vi "João aula 5.vi"() -> ()   [LabVIEW 2024]
uses:
  <vilib>/LabVIEW Open Source Project/Epoch Date & Time/epoch.UNIX/Epoch.UNIX.lvclass
panel:
  out "Potencia ativa C":waveform(dbl)(graph)
  out "Potencia ativa C":waveform(dbl)(graph)
  out "Potencia ativa C":waveform(dbl)
  out "Potencia ativa B":waveform(dbl)(graph)
  out "Potencia ativa B":waveform(dbl)(graph)
  out "Potencia ativa B":waveform(dbl)
  out "Potencia ativa A":waveform(dbl)(graph)
  out "Potencia ativa A":waveform(dbl)(graph)
  in  "stop":bool
  out "Potencia ativa A":waveform(dbl)
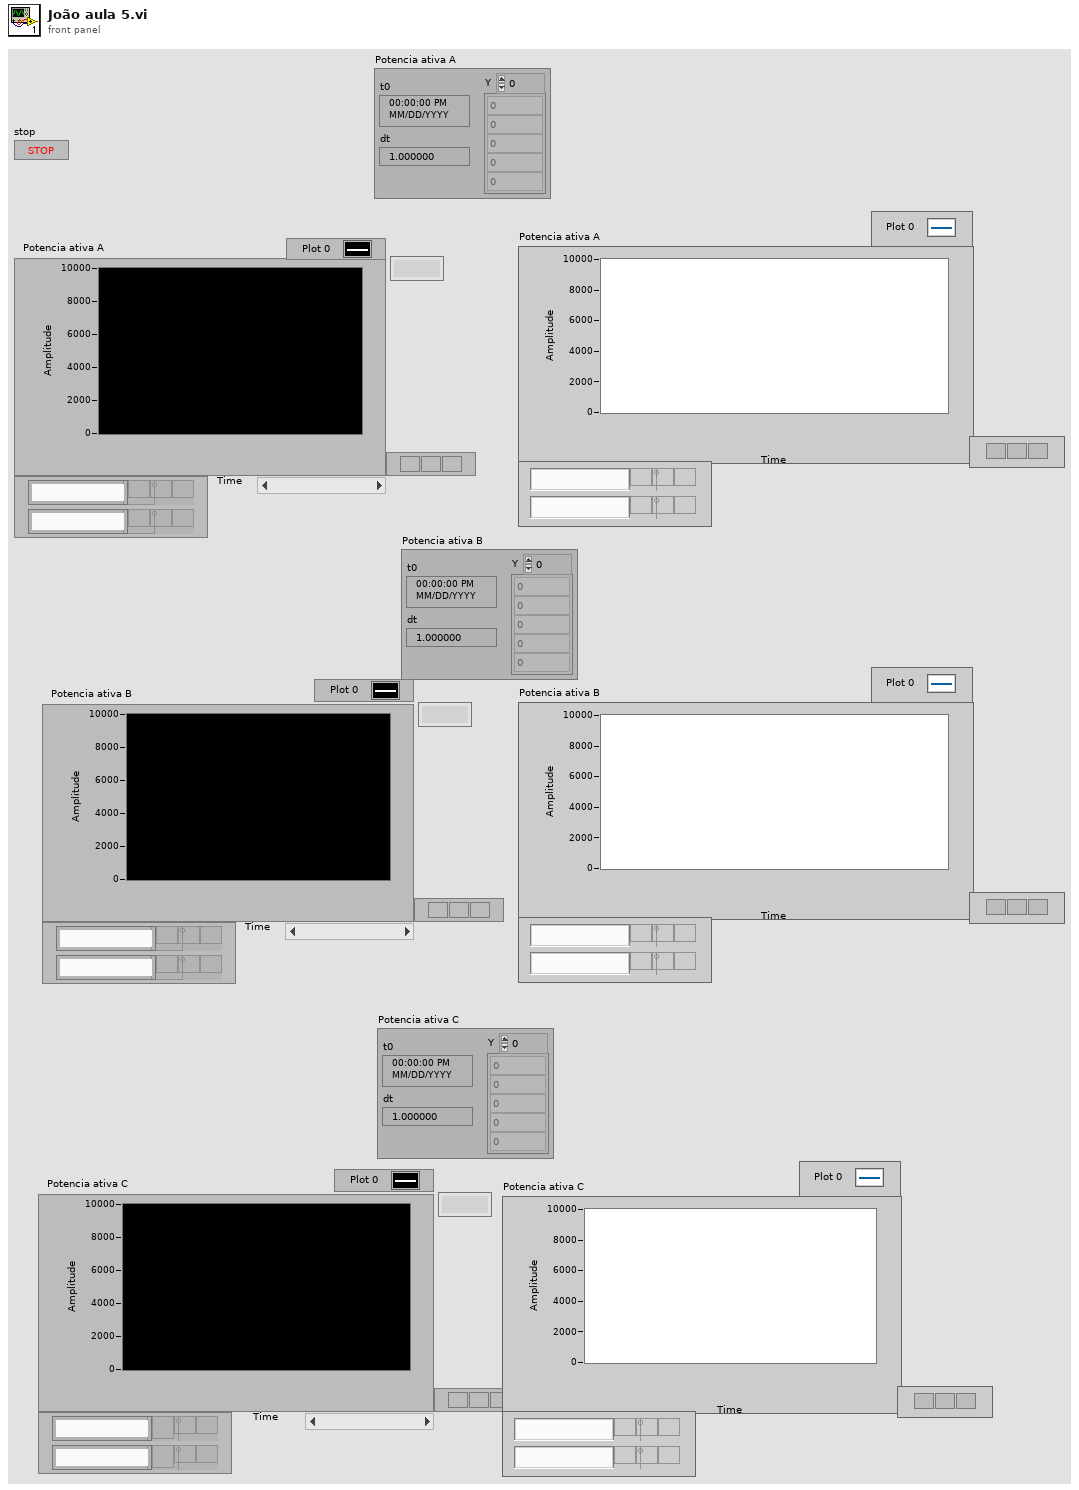
[diagram p1: front panel]
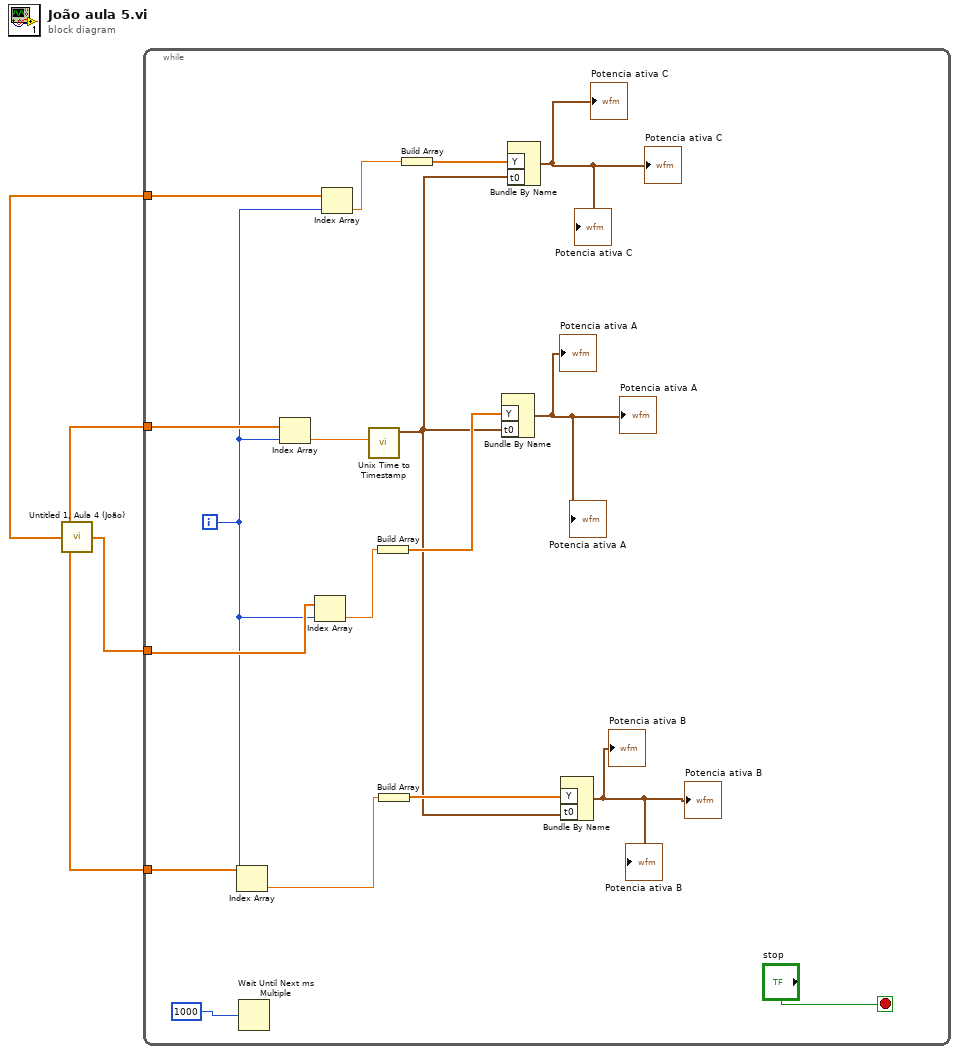
[diagram p0: block diagram]
diagram:
  n1 = call "Untitled 1, Aula 4 (João).vi"() -> ("Potencia ativa A"=w4:dbl[], "Potencia ativa B"=w2:dbl[], "Potencia ativa C"=w1:dbl[], "timestamp"=w3:dbl[])
  n2 = while {
    tunnel: w4 -> [w22]
    tunnel: w3 -> [w21]
    tunnel: w2 -> [w12]
    tunnel: w1 -> [w8]
    i -> [w7]
    stop <- "stop" stop-if-true
    n3 = Index Array(array=w12, index=w7) -> (element=w13:dbl)
    n4 = Wait Until Next ms Multiple(millisecond multiple=u32 1000) -> ()  [unwired: 1 out]
    n5 = Index Array(array=w21, index=w7) -> (element=w20:dbl)
    n6 = Index Array(array=w22, index=w7) -> (element=w18:dbl)
    n7 = Index Array(array=w8, index=w7) -> (element=w9:dbl)
    n8 = call <vilib>:"Unix Time to Timestamp.vi"("Fractional Second"=w20) -> ("Timestamp"=w5:timestamp)  [unwired: 9 in, 1 out]
    n9 = Build Array(w18) -> (w17:dbl[])
    n10 = Build Array(w13) -> (w11:dbl[])
    n11 = Build Array(w9) -> (w6:dbl[])
    n12 = Bundle By Name("Y"=w17, "t0"=w5) -> (→"Potencia ativa A" →"Potencia ativa A" →"Potencia ativa A":waveform(dbl))  [unwired: 1 in]
    n13 = Bundle By Name("Y"=w6, "t0"=w5) -> (→"Potencia ativa C" →"Potencia ativa C" →"Potencia ativa C":waveform(dbl))  [unwired: 1 in]
    n14 = Bundle By Name("Y"=w11, "t0"=w5) -> (→"Potencia ativa B" →"Potencia ativa B" →"Potencia ativa B":waveform(dbl))  [unwired: 1 in]
  }
